vi "Exercise 4.1 - Understanding Property Nodes with Color.vi"() -> ()   [LabVIEW 2012]
panel:
  in  "Visible":bool
  in  "stop":bool
  out "Gauge":dbl(knob) scale=0.0..10.0
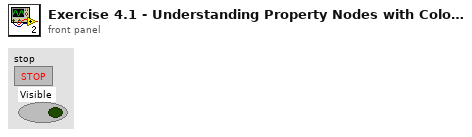
[diagram p1: front panel]
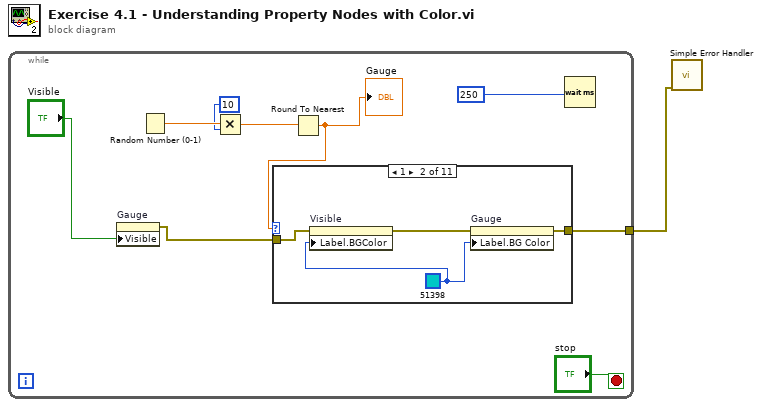
[diagram p0: block diagram]
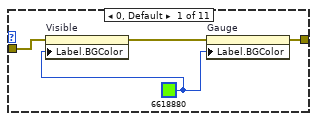
[diagram p2: hidden frame]
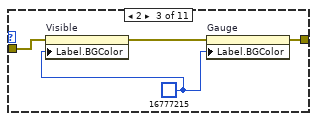
[diagram p3: hidden frame]
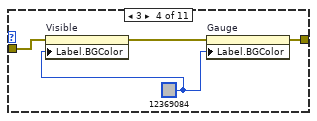
[diagram p4: hidden frame]
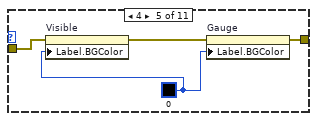
[diagram p5: hidden frame]
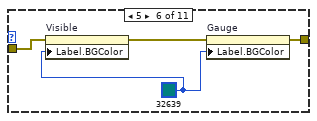
[diagram p6: hidden frame]
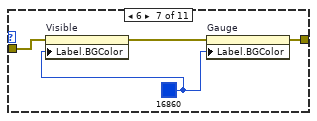
[diagram p7: hidden frame]
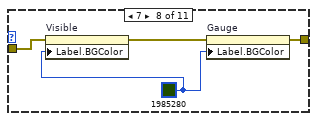
[diagram p8: hidden frame]
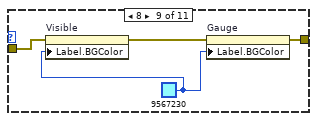
[diagram p9: hidden frame]
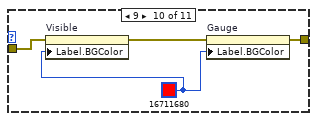
[diagram p10: hidden frame]
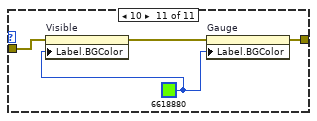
[diagram p11: hidden frame]
diagram:
  n1 = while {
    tunnel: [w5] -> w1
    stop <- "stop" stop-if-true
    n2 = property on="Gauge" class="Knob (strict)"("Visible"="Visible") -> (error out=w7:errorcluster)  [unwired: 2 in, 1 out]
    n3 = Random Number (0-1)() -> (number: 0 to 1=w9:dbl)
    n4 = Multiply(x=w9, y=10 ("Numeric")) -> (x*y=w8:dbl)
    n5 = Round To Nearest(number=w8) -> (nearest integer value=w2:dbl)
    "Gauge" <- w2
    n6 = case shown="1" w2 {
      tunnel: w7 -> [w14 w18 w22 w26 w30 w34 w38 w42 w46 w50 w54]
      tunnel: [w12 w16 w20 w24 w28 w32 w36 w40 w44 w48 w52] -> w5
      frame 0, Default {
        w11 = u32 6618880
        n7 = property on="Visible" class="Bool (strict)"(error in=w14, "Label.BGColor"=w11) -> (error out=w13:errorcluster)  [unwired: 1 in, 1 out]
        n8 = property on="Gauge" class="Knob (strict)"(error in=w13, "Label.BGColor"=w11) -> (error out=w12:errorcluster)  [unwired: 1 in, 1 out]
      }
      frame 1 {
        w15 = u32 51398
        n9 = property on="Visible" class="Bool (strict)"(error in=w18, "Label.BGColor"=w15) -> (error out=w17:errorcluster)  [unwired: 1 in, 1 out]
        n10 = property on="Gauge" class="Knob (strict)"(error in=w17, "Label.BG Color"=w15) -> (error out=w16:errorcluster)  [unwired: 1 in, 1 out]
      }
      frame 2 {
        w19 = u32 16777215
        n11 = property on="Visible" class="Bool (strict)"(error in=w22, "Label.BGColor"=w19) -> (error out=w21:errorcluster)  [unwired: 1 in, 1 out]
        n12 = property on="Gauge" class="Knob (strict)"(error in=w21, "Label.BGColor"=w19) -> (error out=w20:errorcluster)  [unwired: 1 in, 1 out]
      }
      frame 3 {
        w23 = u32 12369084
        n13 = property on="Visible" class="Bool (strict)"(error in=w26, "Label.BGColor"=w23) -> (error out=w25:errorcluster)  [unwired: 1 in, 1 out]
        n14 = property on="Gauge" class="Knob (strict)"(error in=w25, "Label.BGColor"=w23) -> (error out=w24:errorcluster)  [unwired: 1 in, 1 out]
      }
      frame 4 {
        w27 = u32 0
        n15 = property on="Visible" class="Bool (strict)"(error in=w30, "Label.BGColor"=w27) -> (error out=w29:errorcluster)  [unwired: 1 in, 1 out]
        n16 = property on="Gauge" class="Knob (strict)"(error in=w29, "Label.BGColor"=w27) -> (error out=w28:errorcluster)  [unwired: 1 in, 1 out]
      }
      frame 5 {
        w31 = u32 32639
        n17 = property on="Visible" class="Bool (strict)"(error in=w34, "Label.BGColor"=w31) -> (error out=w33:errorcluster)  [unwired: 1 in, 1 out]
        n18 = property on="Gauge" class="Knob (strict)"(error in=w33, "Label.BGColor"=w31) -> (error out=w32:errorcluster)  [unwired: 1 in, 1 out]
      }
      frame 6 {
        w35 = u32 16860
        n19 = property on="Visible" class="Bool (strict)"(error in=w38, "Label.BGColor"=w35) -> (error out=w37:errorcluster)  [unwired: 1 in, 1 out]
        n20 = property on="Gauge" class="Knob (strict)"(error in=w37, "Label.BGColor"=w35) -> (error out=w36:errorcluster)  [unwired: 1 in, 1 out]
      }
      frame 7 {
        w39 = u32 1985280
        n21 = property on="Visible" class="Bool (strict)"(error in=w42, "Label.BGColor"=w39) -> (error out=w41:errorcluster)  [unwired: 1 in, 1 out]
        n22 = property on="Gauge" class="Knob (strict)"(error in=w41, "Label.BGColor"=w39) -> (error out=w40:errorcluster)  [unwired: 1 in, 1 out]
      }
      frame 8 {
        w43 = u32 9567230
        n23 = property on="Visible" class="Bool (strict)"(error in=w46, "Label.BGColor"=w43) -> (error out=w45:errorcluster)  [unwired: 1 in, 1 out]
        n24 = property on="Gauge" class="Knob (strict)"(error in=w45, "Label.BGColor"=w43) -> (error out=w44:errorcluster)  [unwired: 1 in, 1 out]
      }
      frame 9 {
        w47 = u32 16711680
        n25 = property on="Visible" class="Bool (strict)"(error in=w50, "Label.BGColor"=w47) -> (error out=w49:errorcluster)  [unwired: 1 in, 1 out]
        n26 = property on="Gauge" class="Knob (strict)"(error in=w49, "Label.BGColor"=w47) -> (error out=w48:errorcluster)  [unwired: 1 in, 1 out]
      }
      frame 10 {
        w51 = u32 6618880
        n27 = property on="Visible" class="Bool (strict)"(error in=w54, "Label.BGColor"=w51) -> (error out=w53:errorcluster)  [unwired: 1 in, 1 out]
        n28 = property on="Gauge" class="Knob (strict)"(error in=w53, "Label.BGColor"=w51) -> (error out=w52:errorcluster)  [unwired: 1 in, 1 out]
      }
    }
    n29 = Wait (ms)(milliseconds to wait=u32 250 ("millisecond timer value")) -> ()  [unwired: 1 out]
  }
  n30 = call <vilib>:"Simple Error Handler.vi"("error in (no error)"=w1) -> ()  [unwired: 4 in, 5 out]
